vi "Search Direction Constants.vi"() -> (2 "Search Directions":T1[](array[typedef])=[enum."Right", enum."Down", enum."Left", enum."Up"], 3 "Search Direction Cells":T2[](array[typedef]))   [LabVIEW 2019, in "Grassfire Algorithm.lvclass"]
uses:
  Grassfire Algorithm.lvclass
  Index Column Row--cluster.ctl
  Direction--enum.ctl
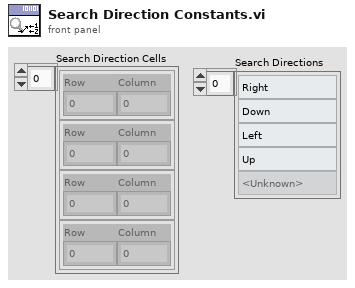
[diagram p1: front panel]
types:
  T1 = typedef "Grassfire Algorithm.lvclass/Direction--enum.ctl" = enum16{"<Unknown>", "Right", "Down", "Left", "Up"}
  T2 = typedef "Grassfire Algorithm.lvclass/Index Column Row--cluster.ctl" = cluster{"Row":i32, "Column":i32}
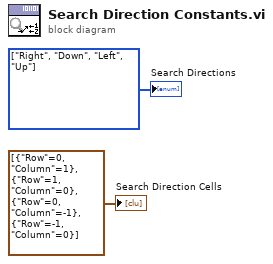
[diagram p0: block diagram]
diagram:
  w1 = T1[] [enum."Right", enum."Down", enum."Left", enum."Up"] items=["<Unknown>", "Right", "Down", "Left", "Up"]
  "Search Direction Cells" <- T2[] [{"Row"=0, "Column"=1}, {"Row"=1, "Column"=0}, {"Row"=0, "Column"=-1}, {"Row"=-1, "Column"=0}]
  "Search Directions" <- w1
